vi "Open File.vi"(8 "error in (no error)":errorcluster, 11 "Spectrum Recorder in":refnum<class "Spectrum Recorder too.lvclass">) -> (0 "error out":errorcluster, 3 "Spectrum Recorder out":refnum<class "Spectrum Recorder too.lvclass">)   [LabVIEW 2016, in "Spectrum Recorder too.lvclass"]
uses:
  Spectrum Recorder too.lvclass
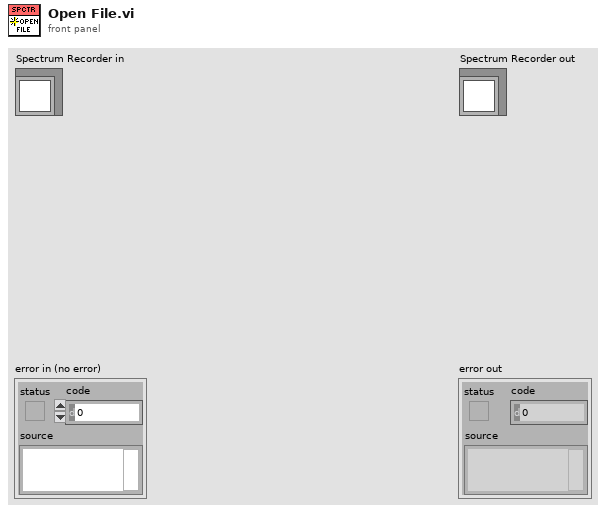
[diagram p1: front panel]
types:
  T1 = typedef "Spectrum Configuration.ctl" = cluster{"Start":dbl, "End":dbl, "Duration":dbl, "Filter time constant":dbl, "Address":string}
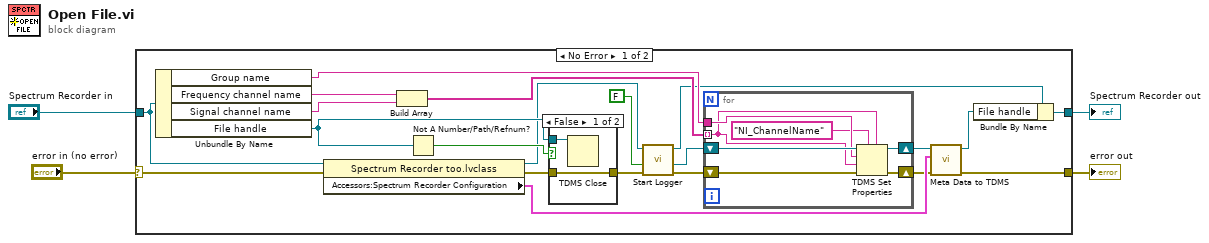
[diagram p0: block diagram]
diagram:
  n1 = case shown="No Error" "error in (no error)" {
    selector: "error in (no error)" -> [w20 w37]
    tunnel: [w11 w37] -> w3
    tunnel: [w23 w36] -> w1
    tunnel: "Spectrum Recorder in" -> [w18 w36]
    frame No Error {
      n2 = Unbundle By Name(w18) -> ("Group name"=w22:string, "Frequency channel name"=w21:string, "Signal channel name"=w16:string, "File handle"=w24:refnum<k34>)
      n3 = property class="Spectrum Recorder too.lvclass"(reference=w18, error in=w20) -> (reference out=w10:refnum<class "Spectrum Recorder too.lvclass">, error out=w19:errorcluster, "Accessors:Spectrum Recorder Configuration"=w13:T1)
      n4 = Build Array(w21, w16) -> (w17:string[])
      n5 = Not A Number/Path/Refnum?(number/path/refnum=w24) -> (NaN/Path/Refnum?=w25:bool)
      n6 = case shown="False" w25 {
        tunnel: w24 -> [w34 _]
        tunnel: w19 -> [w33 w35]
        tunnel: [w33 w35] -> w8
        frame False {
          n7 = TDMS Close(11:w34) -> ()  [unwired: 1 in, 2 out]
        }
        frame True {
        }
      }
      n8 = call-dynamic "Start Logger.vi"("error in (no error)"=w8, "Do not store ref"=FALSE ("Include time"), "Worker in"=w10) -> ("error out"=w6:errorcluster, "tdms ref out"=w5:refnum<k34>, "Worker out"=w9:refnum<class "Spectrum Recorder too.lvclass">)  [unwired: 5 in, 1 out]
      n9 = for {
        tunnel: w22 -> [w30]
        tunnel: w17 -> [w26] mode=indexing
        shift-right: [w31] -> w15
        shift-left: w5 -> [w32]
        shift-right: [w28] -> w12
        shift-left: w6 -> [w29]
        n10 = TDMS Set Properties(5:w26, 7:"NI_ChannelName", 8:w29, 9:w26, 10:w30, 11:w32) -> (0:w28:errorcluster, 3:w31:refnum<k34>)  [unwired: 2 out]
      }
      n11 = call "Meta Data to TDMS.vi"("Error In"=w12, "Value"=w13, "tdms file"=w15) -> ("Error Out"=w11:errorcluster, "tdms file out"=w14:refnum<k34>)  [unwired: 7 in]
      n12 = Bundle By Name(cluster=w9, "File handle"=w14) -> (w23:refnum<class "Spectrum Recorder too.lvclass">)
    }
    frame Error {
    }
  }
  "error out" <- w3
  "Spectrum Recorder out" <- w1
